vi "Cleanup.vi"(10 "Critical Stop?":bool, 11 "Panel Actor in":refnum<class "Panel Actor.lvclass">) -> ()   [LabVIEW 2023, in "Panel Actor.lvlib" / "Panel Actor.lvclass"]
doc: "Throws the \"Stopped\" event and destroys all references.\n\n----\nPlease see the following web address for additional documentation and tutorial information:\nhttp://www.mooregoodideas.com/mgi-panel-manager/\n\nAuthor: Derek Trepanier\n\nCopyright (c) 2018, Moore Good Ideas, Inc.\n\nAll rights reserved.\n\nRedistribution and use in source and binary forms, with or without modification, are permitted provided that the following conditions are met:\n\n * Redistributions of source code must retain the above copyright notice, this list of conditions and the following disclaimer.\n * Redistributions in binary form must reproduce the above copyright notice, this list of conditions and the following disclaimer in the documentation and/or other materials provided with the distribution.\n * Neither the name of Moore Good Ideas, Inc. nor the names of its contributors may be used to endorse or promote products derived from this software without specific prior written permission.\n\nTHIS SOFTWARE IS PROVIDED BY THE COPYRIGHT HOLDERS AND CONTRIBUTORS \"AS IS\" AND ANY EXPRESS OR IMPLIED WARRANTIES, INCLUDING, BUT NOT LIMITED TO, THE IMPLIED WARRANTIES OF MERCHANTABILITY AND FITNESS FOR A PARTICULAR PURPOSE ARE DISCLAIMED. IN NO EVENT SHALL THE COPYRIGHT OWNER OR CONTRIBUTORS BE LIABLE FOR ANY DIRECT, INDIRECT, INCIDENTAL, SPECIAL, EXEMPLARY, OR CONSEQUENTIAL DAMAGES (INCLUDING, BUT NOT LIMITED TO, PROCUREMENT OF SUBSTITUTE GOODS OR SERVICES; LOSS OF USE, DATA, OR PROFITS; OR BUSINESS INTERRUPTION) HOWEVER CAUSED AND ON ANY THEORY OF LIABILITY, WHETHER IN CONTRACT, STRICT LIABILITY, OR TORT (INCLUDING NEGLIGENCE OR OTHERWISE) ARISING IN ANY WAY OUT OF THE USE OF THIS SOFTWARE, EVEN IF ADVISED OF THE POSSIBILITY OF SUCH DAMAGE."
uses:
  Library/Panel Actor.lvclass
  Library/Panel Actor.lvclass/Panel Actor.ctl
  Panel/Panel/Panel.lvclass
  Panel/Panel Helper/Panel Helper.lvclass
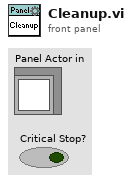
[diagram p1: front panel]
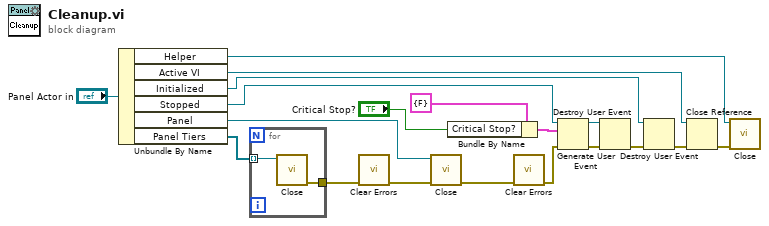
[diagram p0: block diagram]
diagram:
  n1 = Unbundle By Name("Panel Actor in") -> ("Helper"=w18:refnum<class "Panel Helper.lvclass">, "Active VI"=w17:refnum<vi>, "Initialized"=w3:refnum<user-event>, "Stopped"=w11:refnum<user-event>, "Panel"=w10:refnum<class "Panel.lvclass">, "Panel Tiers"=w8:refnum<class "Panel.lvclass">[])
  n2 = for {
    tunnel: w8 -> [w21] mode=indexing
    tunnel: [w20] -> w7
    n3 = call-dynamic "Close.vi"("Panel In"=w21) -> ("Error Out"=w20:errorcluster)  [unwired: 10 in]
  }
  n4 = call <vilib>:"Clear Errors.vi"("error in (no error)"=w7) -> ("error out"=w6:errorcluster)  [unwired: 5 in, 1 out]
  n5 = call-dynamic "Close.vi"("Error In"=w6, "Panel In"=w10) -> ("Error Out"=w15:errorcluster)  [unwired: 9 in]
  n6 = Bundle By Name(cluster=cluster{"Critical Stop?":bool} {"Critical Stop?"=FALSE} ("event data"), "Critical Stop?"="Critical Stop?") -> (w13:cluster{"Critical Stop?":bool})
  n7 = call <vilib>:"Clear Errors.vi"("error in (no error)"=w15) -> ("error out"=w16:errorcluster)  [unwired: 5 in, 1 out]
  n8 = Generate User Event(user event=w11, event data cluster=w13, error in=w16) -> (user event out=w5:refnum<user-event>, error out=w4:errorcluster)  [unwired: 1 in]
  n9 = Destroy User Event(user event=w5, error in=w4) -> (error out=w2:errorcluster)
  n10 = Destroy User Event(user event=w3, error in=w2) -> (error out=w1:errorcluster)
  n11 = Close Reference(reference=w17, error in (no error)=w1) -> (error out=w19:errorcluster)
  n12 = call "Close.vi"("error in (no error)"=w19, "Controller in"=w18) -> ()  [unwired: 9 in, 1 out]
